vi "Update Channels View.vi"(5 "Display State In":T4={"Current Channels Info"=[], "Help Prefix"="", "Max Display Size"=8, "Max Size"=8, "Show Buttons"=TRUE, "Data Valid"=refnum, "Show Range"=FALSE, "Range Items"=[], "Range Index"=[]} caption="State", 7 "Channels In":T1, 8 "error in (no error)":errorcluster, 9 "Move Scorllbar to End":bool, 11 "Channels Reference":refnum<vi>) -> (0 "error out":errorcluster, 1 "Current Index":i32, 4 "Number of Row":i32, 6 "Area Height":u32)   [LabVIEW 2021, in "myRIO Channel List.xctl"]
uses:
  <vilib>/myRIO/Common/Express VI Framework/xctls/myRIO Channel List/myRIO Channel List.xctl
  <vilib>/myRIO/Common/Express VI Framework/xctls/myRIO Channel List/State.ctl
  <vilib>/myRIO/Common/Profile Manager Framework/typedefs/Channel Info.ctl
  <vilib>/myRIO/Common/Express VI Framework/typedefs/Data Validate Ref.ctl
  <vilib>/myRIO/Common/Express VI Framework/xctls/myRIO Channel List/Data.ctl
  <vilib>/myRIO/Common/Express VI Framework/xctls/myRIO Channel List/typedefs/Channel Data.ctl
  <vilib>/myRIO/Common/Express VI Framework/xctls/myRIO Channel List/typedefs/Remove Channel.ctl
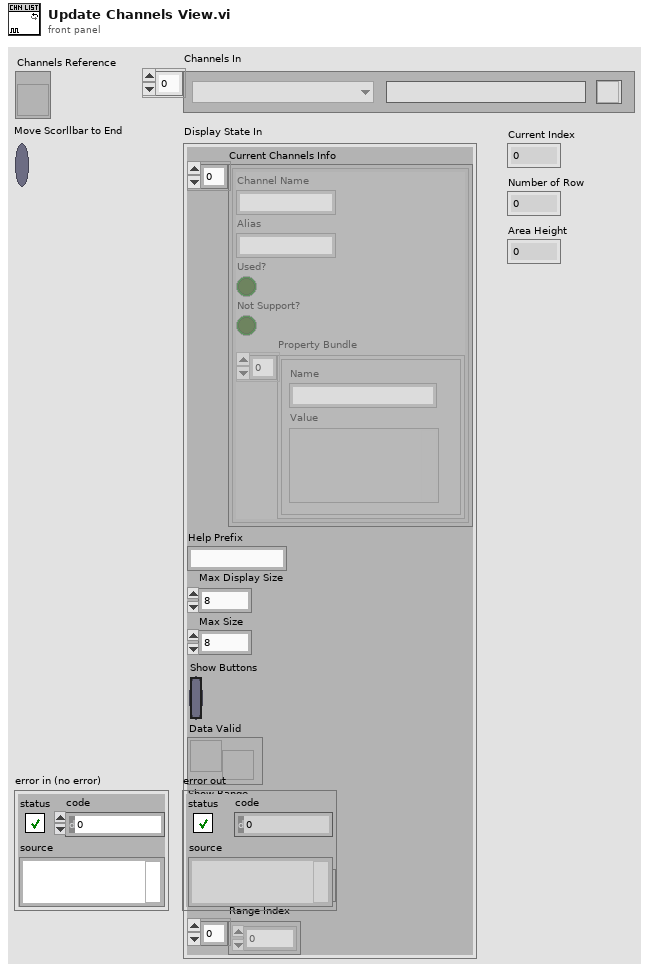
[diagram p1: front panel]
types:
  T1 = typedef "myRIO Channel List.xctl/Data.ctl" = T2[]
  T2 = typedef "myRIO Channel List.xctl/Channel Data.ctl" = cluster{"Channel Name":u16, "Channel Alias":string, "Remove Channel":T3, "Index":i32}
  T3 = typedef "myRIO Channel List.xctl/Remove Channel.ctl" = bool
  T4 = typedef "myRIO Channel List.xctl/State.ctl" = cluster{"Current Channels Info":T5[], "Help Prefix":string, "Max Display Size":i32, "Max Size":i32, "Show Buttons":bool, "Data Valid":T6, "Show Range":bool, "Range Items":string[], "Range Index":i32[]}
  T5 = typedef "Channel Info.ctl" = cluster{"Channel Name":string, "Alias":string, "Used?":bool, "Not Support?":bool, "Property Bundle":cluster{"Name":string, "Value":variant}[]}
  T6 = typedef "Data Validate Ref.ctl" = refnum<user-event>
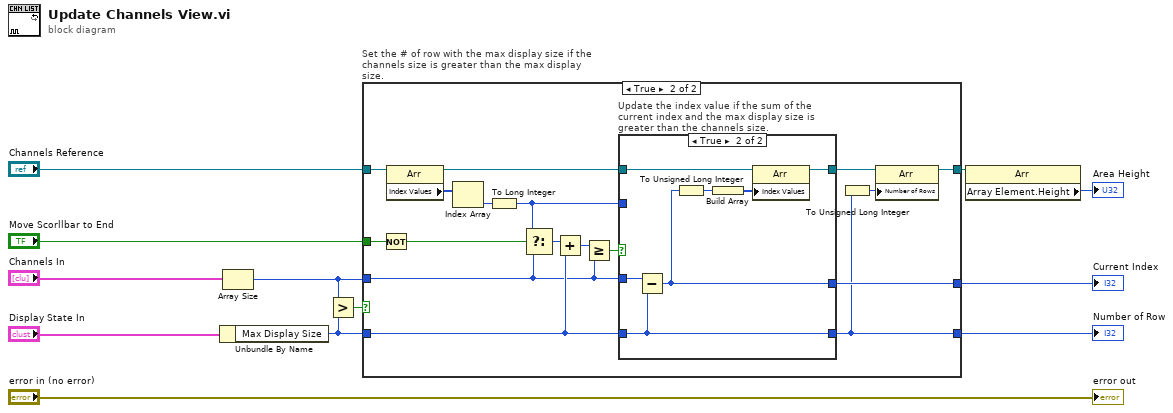
[diagram p0: block diagram]
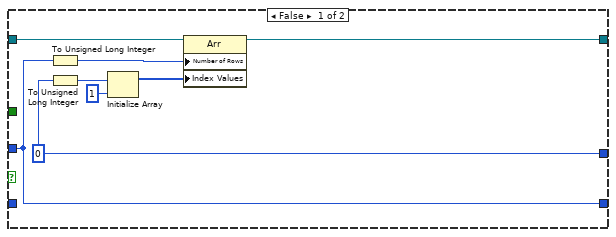
[diagram p2: hidden frame]
diagram:
  n1 = Unbundle By Name("Display State In") -> ("Max Display Size"=w10:i32)
  n2 = Array Size(array="Channels In") -> (size(s)=w11:i32)
  n3 = Greater?(x=w11, y=w10) -> (0:w12:bool)
  n4 = case "Set the # of row with the max display size if the channels size is greater than the max display size." shown="True" w12 {
    tunnel: "Channels Reference" -> [w20 w37]
    tunnel: w11 -> [w14 w25]
    tunnel: w10 -> [_ w32]
    tunnel: [w15 w29] -> w9
    tunnel: [w14 w28] -> w6
    tunnel: [w13 w27] -> w7
    tunnel: "Move Scorllbar to End" -> [_ w22]
    frame False {
      w15 = 0
      n5 = To Unsigned Long Integer(number=w14) -> (unsigned 32bit integer=w19:u32)
      n6 = To Unsigned Long Integer(number=w15) -> (unsigned 32bit integer=w16:u32)
      n7 = Initialize Array(w16, 1 ("dimension size")) -> (w17:u32[])
      n8 = property class="Arr"(reference=w20, "Number of Rows"=w19, "Index Values"=w17) -> (reference out=w13:refnum<vi>)  [unwired: 1 in, 1 out]
    }
    frame True {
      n9 = Not(x=w22) -> (.not. x?=w21:bool)
      n10 = property class="Arr"(reference=w37) -> (reference out=w33:refnum<vi>, "Index Values"=w36:u32[])  [unwired: 1 in, 1 out]
      n11 = Index Array(array=w36) -> (element=w35:u32)  [unwired: 1 in]
      n12 = To Long Integer(number=w35) -> (32bit integer=w24:i32)
      n13 = Select(t=w24, s=w21, f=w25) -> (s? t:f=w23:i32)
      n14 = Add(x=w23, y=w32) -> (x+y=w34:i32)
      n15 = Greater Or Equal?(x=w34, y=w25) -> (x >= y?=w26:bool)
      n16 = case "Update the index value if the sum of the current index and the max display size is greater than the channels size." shown="True" w26 {
        tunnel: w33 -> [w40 w46]
        tunnel: w25 -> [_ w47]
        tunnel: w32 -> [w39 w42]
        tunnel: [w40 w43] -> w31
        tunnel: [w39 w42] -> w28
        tunnel: [w38 w41] -> w29
        tunnel: w24 -> [w38 _]
        frame False {
        }
        frame True {
          n17 = Subtract(x=w47, y=w42) -> (x-y=w41:i32)
          n18 = To Unsigned Long Integer(number=w41) -> (unsigned 32bit integer=w45:u32)
          n19 = Build Array(w45) -> (w44:u32[])
          n20 = property class="Arr"(reference=w46, "Index Values"=w44) -> (reference out=w43:refnum<vi>)  [unwired: 1 in, 1 out]
        }
      }
      n21 = To Unsigned Long Integer(number=w28) -> (unsigned 32bit integer=w30:u32)
      n22 = property class="Arr"(reference=w31, "Number of Rows"=w30) -> (reference out=w27:refnum<vi>)  [unwired: 1 in, 1 out]
    }
  }
  "Current Index" <- w9
  "Number of Row" <- w6
  n23 = property class="Arr"(reference=w7) -> ("Array Element.Height"=→"Area Height":u32)  [unwired: 1 in, 2 out]
  "error out" <- "error in (no error)"
